vi "N Normalize2DGaussianParameters.vi"(1 "best fit parameters IN":dbl[](array[numeric])) -> (0 "best fit parameters OUT":dbl[](array[numeric]))   [LabVIEW 2011]
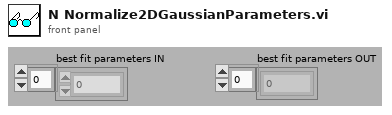
[diagram p1: front panel]
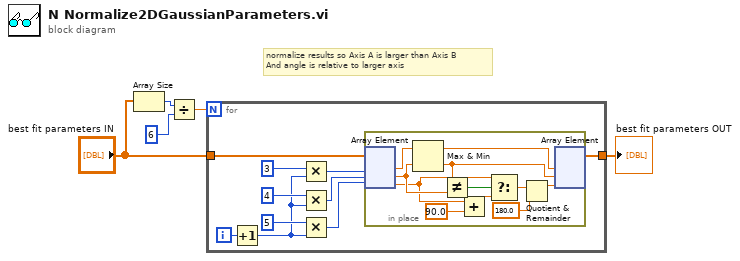
[diagram p0: block diagram]
diagram:
  # "normalize results so Axis A is larger than Axis B\nAnd angle is relative to larger axis"
  n1 = Array Size(array="best fit parameters IN") -> (size(s)=w4:i32)
  n2 = Divide(x=w4, y=6) -> (x/y=w1:dbl)
  n3 = for {
    N: w1 -> [_]
    tunnel: [w15] -> w5
    tunnel: "best fit parameters IN" -> [w14]
    i -> [w13]
    n4 = Increment(x=w13) -> (x+1=w9:i32)
    n5 = Multiply(x=3, y=w9) -> (x*y=w8:i32)
    n6 = Multiply(x=4, y=w9) -> (x*y=w7:i32)
    n7 = Multiply(x=5, y=w9) -> (x*y=w6:i32)
    n8 = in-place {
      n9 = in-place-array #1(w14, w8, w7, w6) -> (w25:dbl, w22:dbl, w18:dbl)
      n10 = Max & Min(x=w25, y=w22) -> (max(x,y)=w24:dbl, min(x,y)=w23:dbl)
      n11 = Not Equal?(x=w23, y=w22) -> (x != y?=w19:bool)
      n12 = Add(x=w18, y=90.0) -> (x+y=w17:dbl)
      n13 = Select(t=w18, s=w19, f=w17) -> (s? t:f=w20:dbl)
      n14 = Quotient & Remainder(x=w20, y=180.0) -> (x-y*floor(x/y)=w26:dbl)  [unwired: 1 out]
      n15 = in-place-array #1(w24, w23, w26) -> (w15:dbl[])  [unwired: 3 out]
    }
  }
  "best fit parameters OUT" <- w5
